vi "Calculate Position Relative To Owner.vi"(11 "Zap Sat in":refnum<class "Zap Sat.lvclass">) -> (3 "Position":refnum<class "Vector 2D.lvclass">)   [LabVIEW 2021, in "Zap Sat.lvclass"]
uses:
  Zap Sat.lvclass
  Re-use Libraries/Vector 2D/Vector 2D.lvclass
  Zap Sat.lvclass/Zap Sat.ctl
  Globals.vi
  Element/Element.lvclass
panel:
  in  "Radius":sgl(slide)=200.0 scale=0.0..400.0
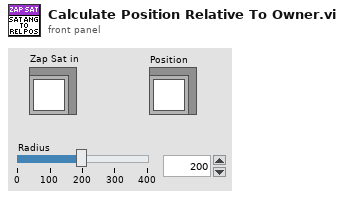
[diagram p1: front panel]
types:
  T1 = typedef "Element.lvclass/Player Type.ctl" = enum16{"Neutral", "Player 1", "Player 2"}
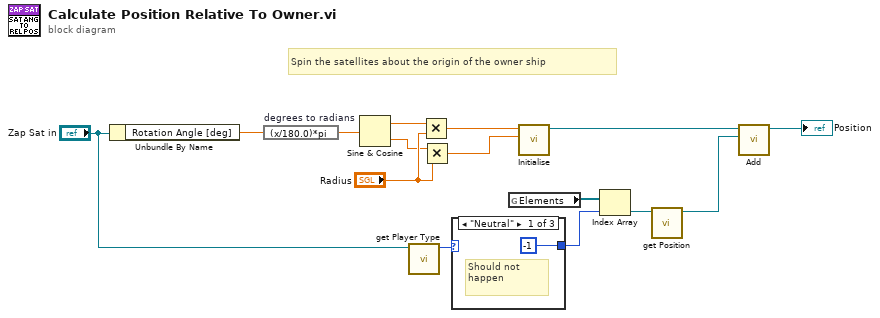
[diagram p0: block diagram]
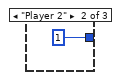
[diagram p2: hidden frame]
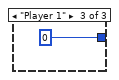
[diagram p3: hidden frame]
diagram:
  # "Spin the satellites about the origin of the owner ship"
  n1 = Unbundle By Name("Zap Sat in") -> ("Rotation Angle [deg]"=w9:sgl)
  n2 = expression code="(x/180.0)*pi" "degrees to radians"(w9) -> (w12:sgl)
  n3 = Sine & Cosine(0:w12) -> (1:w14:sgl, 2:w13:sgl)
  n4 = call "get Player Type.vi"("Element in"="Zap Sat in") -> ("Player Type"=w2:T1)  [unwired: 10 in]
  n5 = Multiply(x=w14, y="Radius") -> (x*y=w11:sgl)
  n6 = Multiply(x=w13, y="Radius") -> (x*y=w10:sgl)
  n7 = case shown="\"Neutral\"" w2 {
    tunnel: [-1 1 0] -> w1
    frame "Neutral" {
      # "Should not happen"
    }
    frame "Player 2" {
    }
    frame "Player 1" {
    }
  }
  n8 = global read "Globals.vi" "Elements"() -> (w7:refnum<class "Element.lvclass">[])
  n9 = call "Initialise.vi"("y"=w10, "x"=w11) -> ("Vector 2D out"=w6:refnum<class "Vector 2D.lvclass">)  [unwired: 9 in]
  n10 = Index Array(array=w7, index=w1) -> (element=w8:refnum<class "Element.lvclass">)
  n11 = call "get Position.vi"("Element in"=w8) -> ("Position"=w5:refnum<class "Vector 2D.lvclass">)  [unwired: 10 in]
  n12 = call "Add.vi"("B"=w5, "A"=w6) -> ("A+B"=→"Position":refnum<class "Vector 2D.lvclass">)  [unwired: 9 in]
